vi "correspondence table extrapolator.vi"(2 "Volts":dbl format="%.2f", 3 "correspondence table":cluster{"physical units":dbl, "volts":dbl}[](array[cluster]) {"volts" format="%.2f"; "physical units" format="%.2f"}) -> (0 "scaled":dbl format="%.2f", 1 "comparison":enum16{"less than", "in range", "greater than"}(ring))   [LabVIEW 2019]
uses:
  <vilib>/Analysis/NI_AALPro.lvlib
panel:
  # "volts must be increasing with index"
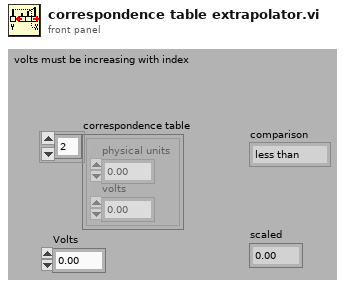
[diagram p1: front panel]
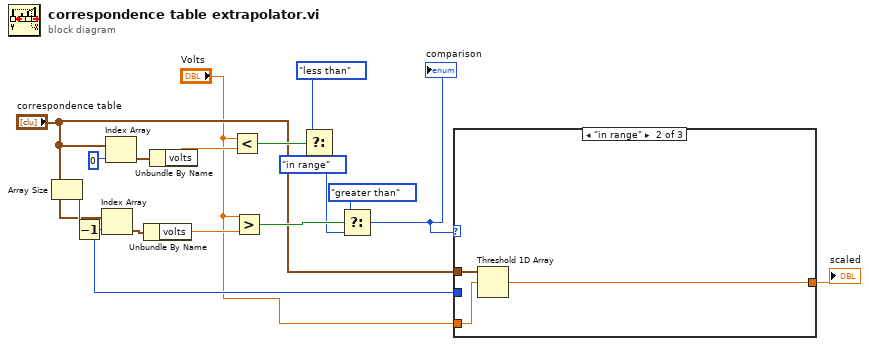
[diagram p0: block diagram]
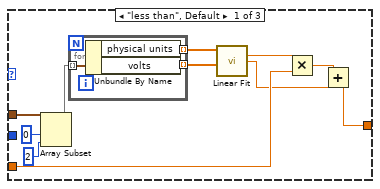
[diagram p2: hidden frame]
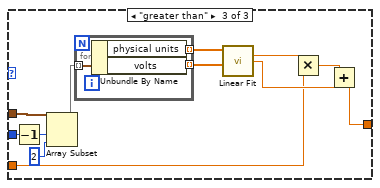
[diagram p3: hidden frame]
diagram:
  n1 = Array Size(array="correspondence table") -> (size(s)=w16:i32)
  n2 = Decrement(x=w16) -> (x-1=w15:i32)
  n3 = Index Array(array="correspondence table", index=w15) -> (element=w13:cluster{"physical units":dbl, "volts":dbl})
  n4 = Index Array(array="correspondence table", index=0 ("Index")) -> (element=w14:cluster{"physical units":dbl, "volts":dbl})
  n5 = Unbundle By Name(w13) -> ("volts"=w11:dbl)
  n6 = Unbundle By Name(w14) -> ("volts"=w12:dbl)
  n7 = Less?(x="Volts", y=w12) -> (x < y?=w10:bool)
  n8 = Greater?(x="Volts", y=w11) -> (0:w9:bool)
  n9 = Select(t=enum16{"less than", "in range", "greater than"}."less than" ("comparison"), s=w10, f=enum16{"less than", "in range", "greater than"}."in range" ("comparison")) -> (s? t:f=w8:enum16{"less than", "in range", "greater than"})
  n10 = Select(t=enum16{"less than", "in range", "greater than"}."greater than" ("comparison"), s=w9, f=w8) -> (s? t:f=w7:enum16{"less than", "in range", "greater than"})
  "comparison" <- w7
  n11 = case shown="\"in range\"" w7 {
    tunnel: "correspondence table" -> [w28 w34 w39]
    tunnel: "Volts" -> [w21 w33 w37]
    tunnel: [w18 w32 w38] -> w2
    tunnel: w15 -> [_ _ w36]
    frame "less than", Default {
      n12 = Array Subset(array=w28, index=0 ("Array Index"), length=2 ("Array Length")) -> (w25:cluster{"physical units":dbl, "volts":dbl}[])
      n13 = for {
        tunnel: w25 -> [w31] mode=indexing
        tunnel: [w30] -> w24 mode=indexing
        tunnel: [w29] -> w23 mode=indexing
        n14 = Unbundle By Name(w31) -> ("physical units"=w30:dbl, "volts"=w29:dbl)
      }
      n15 = call <vilib>:"Linear Fit.vi"("Y"=w24, "X"=w23) -> ("slope"=w22:dbl, "intercept"=w19:dbl)  [unwired: 9 in, 3 out]
      n16 = Multiply(x=w22, y=w21) -> (x*y=w20:dbl)
      n17 = Add(x=w20, y=w19) -> (x+y=w18:dbl)
    }
    frame "in range" {
      n18 = Threshold 1D Array(2:w33, 3:w34) -> (0:w32:dbl)  [unwired: 1 in]
    }
    frame "greater than" {
      n19 = Decrement(x=w36) -> (x-1=w35:i32)
      n20 = Array Subset(array=w39, index=w35, length=2 ("Array Length")) -> (w45:cluster{"physical units":dbl, "volts":dbl}[])
      n21 = for {
        tunnel: w45 -> [w49] mode=indexing
        tunnel: [w48] -> w44 mode=indexing
        tunnel: [w47] -> w43 mode=indexing
        n22 = Unbundle By Name(w49) -> ("physical units"=w48:dbl, "volts"=w47:dbl)
      }
      n23 = call <vilib>:"Linear Fit.vi"("Y"=w44, "X"=w43) -> ("slope"=w42:dbl, "intercept"=w40:dbl)  [unwired: 9 in, 3 out]
      n24 = Multiply(x=w42, y=w37) -> (x*y=w41:dbl)
      n25 = Add(x=w41, y=w40) -> (x+y=w38:dbl)
    }
  }
  "scaled" <- w2
